vi "api_mqttPublish.vi"(4 "messageID":u16, 6 "connMeta":T1, 8 "error in (no error)":errorcluster, 9 "value":string, 10 "topic":string, 11 "mqtt in":refnum<class "mqtt.lvclass">) -> (0 "error out":errorcluster, 3 "mqtt out":refnum<class "mqtt.lvclass">)   [LabVIEW 2020, in "mqtt.lvclass"]
uses:
  mqtt.lvclass
  mqttTypedef/mqttRXdataCluster.ctl
  mqttTypedef/mqttFixedHeaderResponse.ctl
  mqttTypedef/mqttQOSlevel.ctl
  mqttTypedef/mqttMessageType.ctl
  mqttTypedef/mqttConnectionMeta.ctl
  mqttCmd/mqttCmdPublish/mqttCmdPublish.lvclass
  C:/Projects/Libraries/Gore SM 2020/mqtt-LabVIEW/src/class/mqtt/mqttCmd/mqttCmd.lvclass
panel:
  out "notification":T3
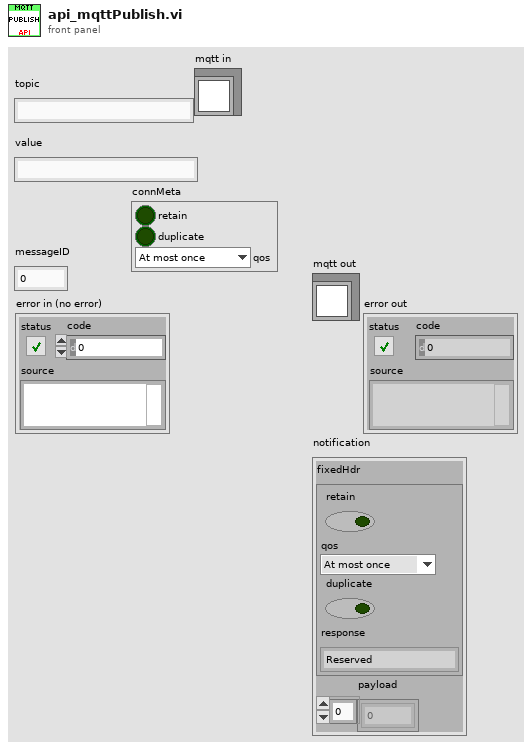
[diagram p1: front panel]
types:
  T1 = typedef "mqttConnectionMeta.ctl" = cluster{"retain":bool, "duplicate":bool, "qos":T2}
  T2 = typedef "mqttQOSlevel.ctl" = enum8{"At most once", "At least once", "Exactly once", "Reserved"}
  T3 = typedef "mqttRXdataCluster.ctl" = cluster{"fixedHdr":T4, "payload":u8[]}
  T4 = typedef "mqttFixedHeaderResponse.ctl" = cluster{"retain":bool, "qos":T2, "duplicate":bool, "response":T5}
  T5 = typedef "mqttMessageType.ctl" = enum32{"Reserved", "CONNECT", "CONNACK", "PUBLISH", "PUBACK", "PUBREC", "PUBREL", "PUBCOMP", "SUBSCRIBE", "SUBACK", "UNSUBSCRIBE", "UNSUBACK", "PINGREQ", "PINGRESP", "DISCONNECT", "Reserved2"}
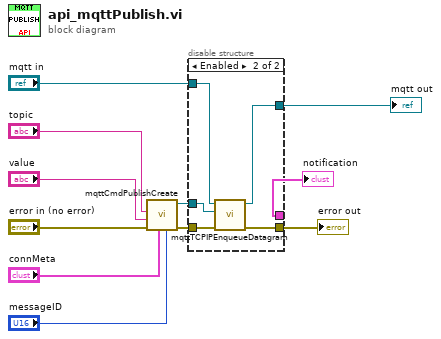
[diagram p0: block diagram]
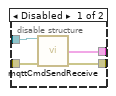
[diagram p2: hidden frame]
diagram:
  n1 = call "mqttCmdPublishCreate.vi"("messageID"="messageID", "connMeta"="connMeta", "error in (no error)"="error in (no error)", "value"="value", "topic"="topic") -> ("error out"=w5:errorcluster, "mqttCmdPublish out"=w4:refnum<class "mqttCmdPublish.lvclass">)  [unwired: 5 in]
  n2 = disable-structure shown="Enabled" {
    disable-tunnel: [w15 _] -> w10
    disable-tunnel: [w14 w17] -> w9
    disable-tunnel: w5 -> [w13 w18]
    disable-tunnel: w4 -> [w12 w20]
    disable-tunnel: "mqtt in" -> [_ w19]
    disable-tunnel: [_ w16] -> w1
    frame Disabled {
      n3 = call "mqttCmdSendReceive.vi"("mqttConnect in"=w12, "error in (no error)"=w13) -> ("notification"=w15:T3, "error out"=w14:errorcluster)  [unwired: 10 in, 2 out]
    }
    frame Enabled {
      n4 = call "mqttTCPIPEnqueueDatagram.vi"("error in (no error)"=w18, "mqttCmd"=w20, "mqtt in"=w19) -> ("error out"=w17:errorcluster, "mqtt out"=w16:refnum<class "mqtt.lvclass">)  [unwired: 7 in]
    }
  }
  "error out" <- w9
  "notification" <- w10
  "mqtt out" <- w1
